vi "Locate HPRF Spark Mark II.vi"(5 "Channel Data":dbl[][](array[numeric]), 9 "Correlation Window Offset (S)":i32, 11 "Correlation Window Duration (S)":i32, 12 "Microphone Coordinates (cm, rad)":cluster{"r":dbl, "theta":dbl}[](array[cluster])) -> (8 "Coordinates (cm, rad, cm)":cluster{sgl, sgl, sgl})   [LabVIEW 2013]
uses:
  <vilib>/Analysis/NI_AALPro.lvlib
  <vilib>/Analysis/2dsp.llb/1D Cross Correlation (DBL).vi
panel:
  out "Endcap Signals Cross Correlation":dbl[](graph)
  # "x"
  # "y"
  # "z"
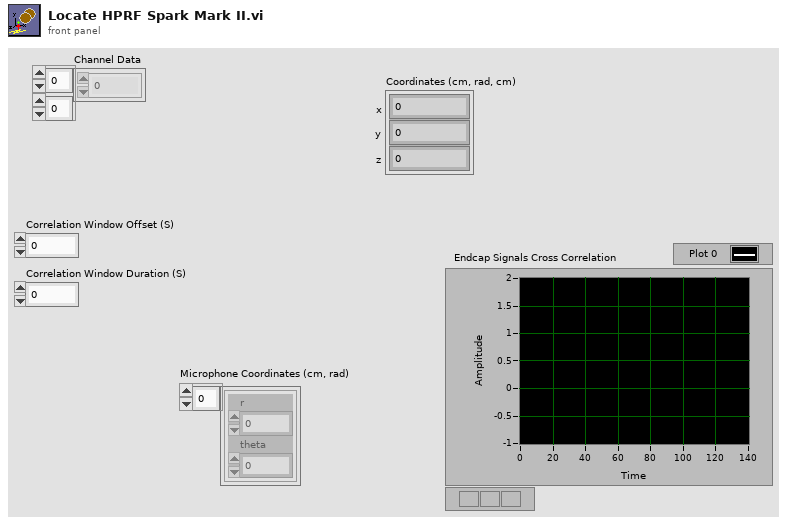
[diagram p1: front panel]
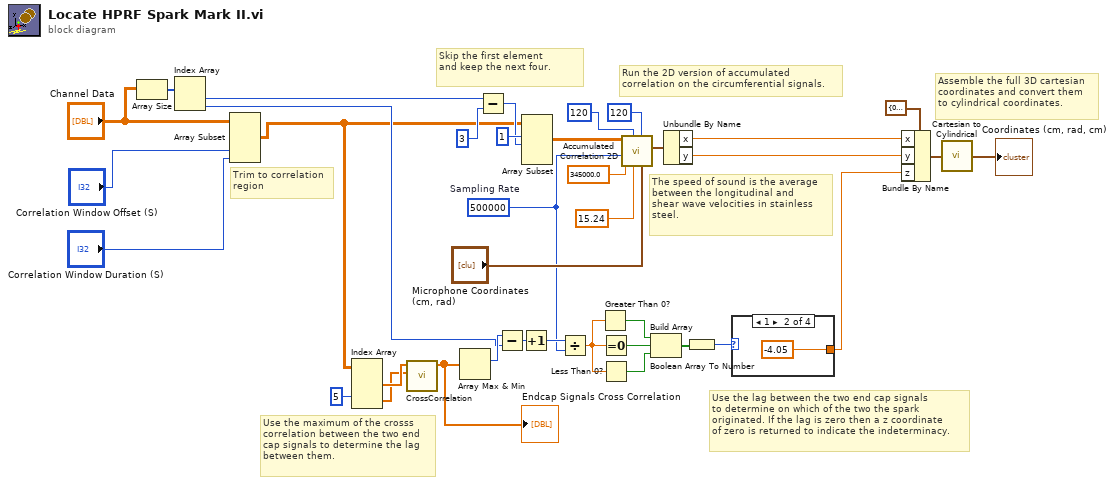
[diagram p0: block diagram]
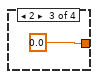
[diagram p3: hidden frame]
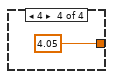
[diagram p4: hidden frame]
diagram:
  w16 = 500000  # Sampling Rate
  # "The speed of sound is the average\nbetween the longitudinal and\nshear wave velocities in stainless\nsteel."
  # "Assemble the full 3D cartesian\ncoordinates and convert them\nto cylindrical coordinates."
  # "Use the lag between the two end cap signals\nto determine on which of the two the spark\noriginated. If the lag is zero then a z coordinate\nof zero is returned to indicate the indeterminacy."
  # "Use the maximum of the crosss\ncorrelation between the two end\ncap signals to determine the lag\nbetween them."
  # "Run the 2D version of accumulated\ncorrelation on the circumferential signals."
  # "Trim to correlation\nregion"
  # "Skip the first element\nand keep the next four."
  n1 = Array Size(array="Channel Data") -> (size(s)=w36:i32[])
  n2 = Index Array(array=w36) -> (element #1=w23:i32, element #2=w17:i32)  [unwired: 2 in]
  n3 = Array Subset(array="Channel Data", index (col)="Correlation Window Offset (S)", length (col)="Correlation Window Duration (S)") -> (w3:dbl[][])  [unwired: 2 in]
  n4 = Index Array(array=w3, index (row) #2=5 ("index")) -> (element #1=w14:dbl[], element #2=w13:dbl[])  [unwired: 3 in]
  n5 = call-poly <vilib>:"CrossCorrelation.vi"("Y"=w13, "X"=w14) -> ("Rxy"=w5:dbl[])  [unwired: 8 in, 1 out]
  "Endcap Signals Cross Correlation" <- w5
  n6 = Array Max & Min(array=w5) -> (max index (indices)=w18:i32)  [unwired: 3 out]
  n7 = Subtract(x=w23, y=3 ("index")) -> (x-y=w21:i32)
  n8 = Subtract(x=w18, y=w17) -> (x-y=w20:i32)
  n9 = Increment(x=w20) -> (x+1=w19:i32)
  n10 = Array Subset(array=w3, index (row)=1 ("index"), length (row)=w21) -> (w35:dbl[][])  [unwired: 2 in]
  n11 = Divide(x=w19, y=w16) -> (x/y=w12:dbl)
  n12 = Greater Than 0?(x=w12) -> (x > 0?=w11:bool)
  n13 = Equal To 0?(x=w12) -> (x = 0?=w10:bool)
  n14 = Less Than 0?(x=w12) -> (x < 0?=w9:bool)
  n15 = call "Accumulated Correlation 2D.vi"("Microphone Coordinates (cm, rad)"="Microphone Coordinates (cm, rad)", "Ny"=120 ("Ntheta"), "Radius (cm)"=15.24, "Nx"=120 ("Nr"), "Sound Velocity (cm/s)"=345000.0, "Sampling Rate"=w16, "Waveforms"=w35) -> ("Source Coordinates (cm, cm)"=w29:cluster{"x":dbl, "y":dbl})  [unwired: 4 in]
  n16 = Build Array(w11, w10, w9) -> (w8:bool[])
  n17 = Unbundle By Name(w29) -> ("x"=w28:dbl, "y"=w25:dbl)
  n18 = Boolean Array To Number(Boolean array=w8) -> (number=w7:u32)
  n19 = case shown="1" w7 {
    tunnel: [_ -4.05 ("z") 0.0 ("z") 4.05 ("z")] -> w6
    frame 0, Default {
    }
    frame 1 {
    }
    frame 2 {
    }
    frame 4 {
    }
  }
  n20 = Bundle By Name(cluster=cluster{"x":dbl, "y":dbl, "z":dbl} {"x"=0.0, "y"=0.0, "z"=0.0} ("Cartesian\nCoordinates"), "x"=w28, "y"=w25, "z"=w6) -> (w26:cluster{"x":dbl, "y":dbl, "z":dbl})
  n21 = call "Cartesian to Cylindrical.vi"("Cartesian\nCoordinates"=w26) -> ("Cylindrical\nCoordinates"=→"Coordinates (cm, rad, cm)":cluster{"r":dbl, "theta":dbl, "z":dbl})  [unwired: 4 in]
